vi "Read SelectionMode.vi"(8 "error in (no error)":errorcluster, 11 "Msg_Error.lvclass in":refnum<class "ListSelection.lvclass">) -> (0 "error out":errorcluster, 2 "Selection Mode":T1, 3 "Msg_Error.lvclass out":refnum<class "ListSelection.lvclass">)   [LabVIEW 2012, in "ListSelection.lvlib" / "ListSelection.lvclass"]
uses:
  ListSelection.lvclass
  Selection Mode.ctl
  ListSelection.lvclass/ListSelection.ctl
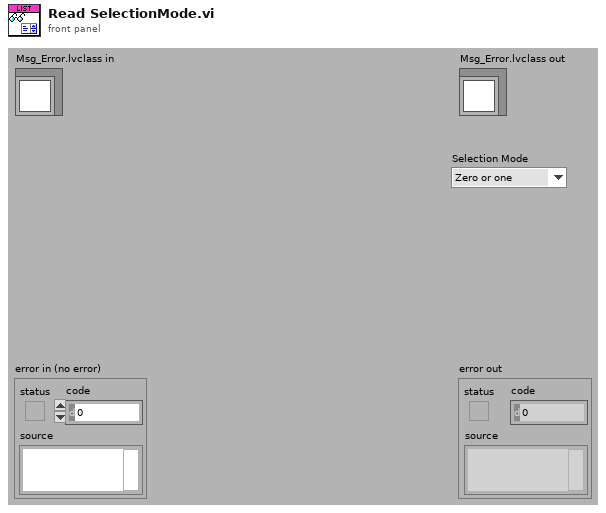
[diagram p1: front panel]
types:
  T1 = typedef "ListSelection.lvlib/ListSelection.lvclass/Selection Mode.ctl" = enum16{"Zero or one", "One", "Zero or more", "One or more"}
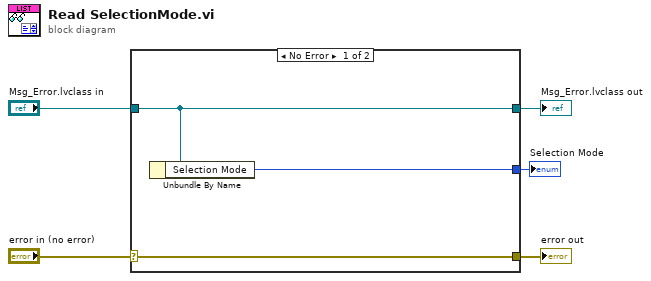
[diagram p0: block diagram]
diagram:
  n1 = case shown="No Error" "error in (no error)" {
    selector: "error in (no error)" -> [w8 w9]
    tunnel: [w8 w9] -> w4
    tunnel: [w7 w10] -> w2
    tunnel: "Msg_Error.lvclass in" -> [w7 w10]
    tunnel: [w6 _] -> w1
    frame No Error {
      n2 = Unbundle By Name(w7) -> ("Selection Mode"=w6:T1)
    }
    frame Error {
    }
  }
  "error out" <- w4
  "Msg_Error.lvclass out" <- w2
  "Selection Mode" <- w1
